vi "WeatherMapAPI_CurrentWeather-ParseResponseJSON.vi"(11 "API JSON Response":string) -> (3 "WeatherMap Current Weather Data":T1)   [LabVIEW 2021]
panel:
  out "Array":string[](array[string])
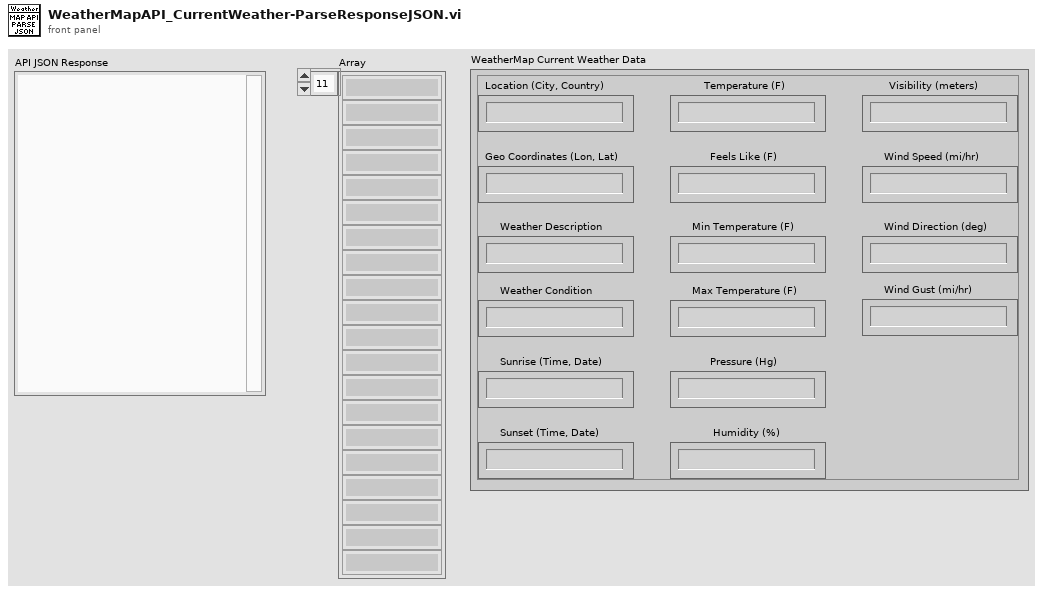
[diagram p1: front panel]
types:
  T1 = cluster{"Location (City, Country)":string, "Geo Coordinates (Lon, Lat)":string, "Weather Description ":string, "Weather Condition":string, "Temperature (F)":string, "Feels Like (F)":string, "Min Temperature (F)":string, "Max Temperature (F)":string, "Pressure (Hg) ":string, "Humidity (%)":string, "Visibility (meters)":string, "Wind Speed (mi/hr)":string, "Wind Direction (deg)":string, "Sunrise (Time, Date)":string, "Sunset (Time, Date)":string, "Wind Gust (mi/hr) ":string}
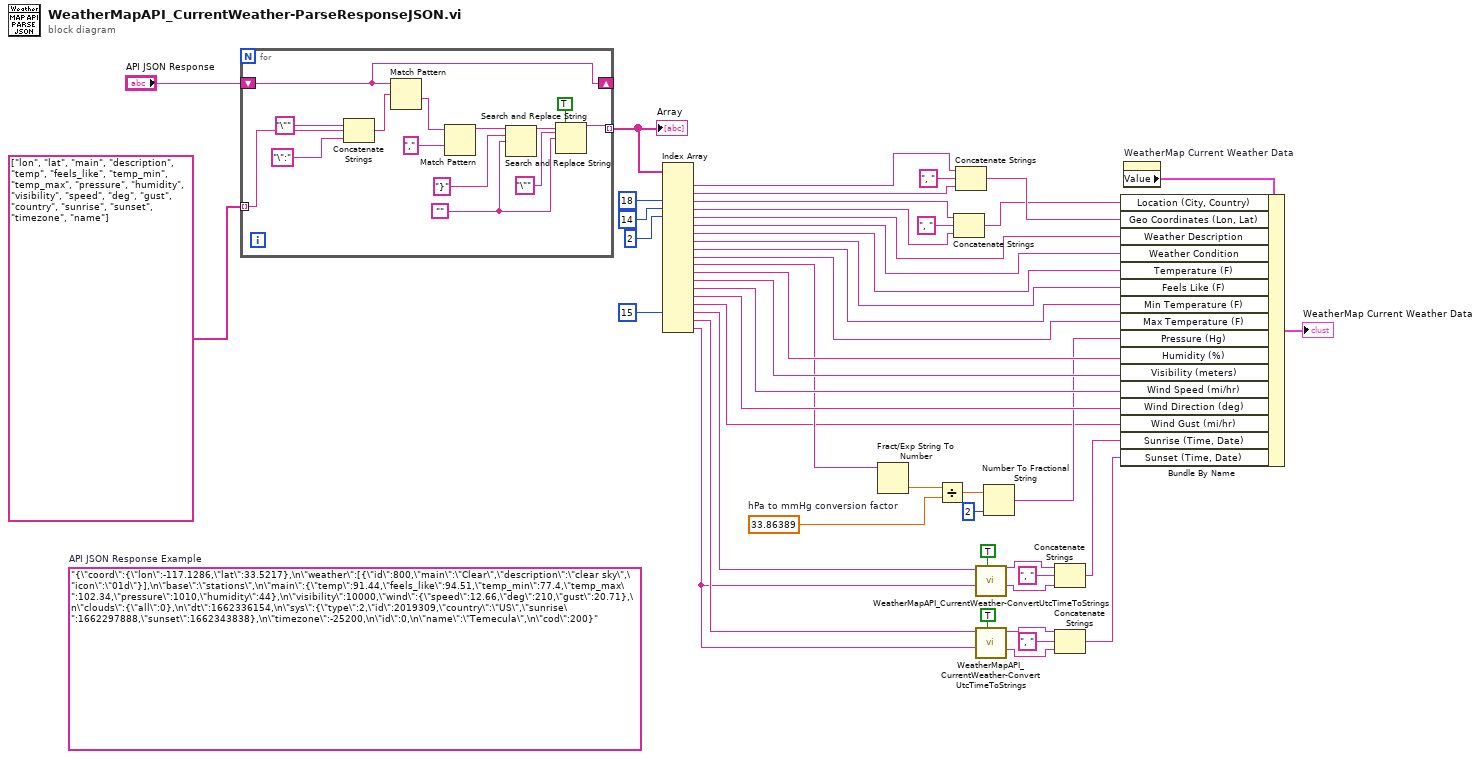
[diagram p0: block diagram]
diagram:
  w13 = 33.86389  # hPa to mmHg conversion factor
  (unwired) "{\"coord\":{\"lon\":-117.1286,\"lat\":33.5217},\n\"weather\":[{\"id\":800,\"main\":\"Clear\",\"description\":\"clear sky\",\"icon\":\"01d\"}],\n\"base\":\"stations\",\n\"main\":{\"temp\":91.44,\"feels_like\":94.51,\"temp_min\":77.4,\"temp_max\":102.34,\"pressure\":1010,\"humidity\":44},\n\"visibility\":10000,\"wind\":{\"speed\":12.66,\"deg\":210,\"gust\":20.71},\n\"clouds\":{\"all\":0},\n\"dt\":1662336154,\n\"sys\":{\"type\":2,\"id\":2019309,\"country\":\"US\",\"sunrise\":1662297888,\"sunset\":1662343838},\n\"timezone\":-25200,\n\"id\":0,\n\"name\":\"Temecula\",\n\"cod\":200}"  # API JSON Response Example
  n1 = for {
    shift-right: [w48] -> _
    shift-left: "API JSON Response" -> [w48]
    tunnel: string[] ["lon", "lat", "main", "description", "temp", "feels_like", "temp_min", "temp_max", "pressure", "humidity", "visibility", "speed", "deg", "gust", "country", "sunrise", "sunset", "timezone", "name"] -> [w58] mode=indexing
    tunnel: [w50] -> w45 mode=indexing
    w53 = ""
    n2 = Concatenate Strings("\"" ("regular expression"), w58, "\":" ("regular expression")) -> (w57:string)
    n3 = Match Pattern(string=w48, regular expression=w57) -> (after substring=w49:string)  [unwired: 1 in, 3 out]
    n4 = Match Pattern(string=w49, regular expression=",") -> (before substring=w55:string)  [unwired: 1 in, 3 out]
    n5 = Search and Replace String(input string=w55, search string="}", replace string=w53) -> (result string=w54:string)  [unwired: 5 in, 3 out]
    n6 = Search and Replace String(replace all?=TRUE ("replace all? (F)"), input string=w54, search string="\"", replace string=w53) -> (result string=w50:string)  [unwired: 4 in, 3 out]
  }
  "Array" <- w45
  n7 = Index Array(array=w45, index #3=18 ("index"), index #4=14 ("index"), index #5=2 ("index"), index #17=15 ("index")) -> (element #1=w43:string, element #2=w42:string, element #3=w37:string, element #4=w36:string, element #5=w31:string, element #6=w30:string, element #7=w29:string, element #8=w28:string, element #9=w27:string, element #10=w26:string, element #11=w8:string, element #12=w25:string, element #13=w24:string, element #14=w23:string, element #15=w22:string, element #16=w5:string, element #17=w3:string, element #18=w2:string, element #19=w1:string)  [unwired: 15 in]
  n8 = Fract/Exp String To Number(string=w8) -> (number=w9:dbl)  [unwired: 3 in, 1 out]
  n9 = Divide(x=w9, y=w13) -> (x/y=w12:dbl)
  n10 = Concatenate Strings(w37, ", " ("regular expression"), w36) -> (w35:string)
  n11 = Concatenate Strings(w43, ", " ("regular expression"), w42) -> (w39:string)
  n12 = call "WeatherMapAPI_CurrentWeather-ConvertUtcTimeToStrings.vi"("1Hr Adjust - Subtract"=TRUE, "Offset from UTC"=w1, "Sunrise/Sunset time, unix, UTC"=w3) -> ("Date"=w18:string, "Time"=w17:string)  [unwired: 7 in]
  n13 = call "WeatherMapAPI_CurrentWeather-ConvertUtcTimeToStrings.vi"("1Hr Adjust - Subtract"=TRUE, "Offset from UTC"=w1, "Sunrise/Sunset time, unix, UTC"=w2) -> ("Date"=w14:string, "Time"=w15:string)  [unwired: 7 in]
  n14 = Number To Fractional String(number=w12, precision (6)=i16 2) -> (F-format string=w10:string)  [unwired: 2 in]
  n15 = Concatenate Strings(w17, ", " ("regular expression"), w18) -> (w6:string)
  n16 = Concatenate Strings(w15, ", " ("regular expression"), w14) -> (w7:string)
  n17 = property on="WeatherMap Current Weather Data" class="Clust (strict)"() -> ("Value"=w40:T1)  [unwired: 2 in, 2 out]
  n18 = Bundle By Name(cluster=w40, "Location (City, Country)"=w35, "Geo Coordinates (Lon, Lat)"=w39, "Weather Description"=w31, "Weather Condition"=w30, "Temperature (F)"=w29, "Feels Like (F)"=w28, "Min Temperature (F)"=w27, "Max Temperature (F)"=w26, "Pressure (Hg)"=w10, "Humidity (%)"=w25, "Visibility (meters)"=w24, "Wind Speed (mi/hr)"=w23, "Wind Direction (deg)"=w22, "Wind Gust (mi/hr)"=w5, "Sunrise (Time, Date)"=w6, "Sunset (Time, Date)"=w7) -> (→"WeatherMap Current Weather Data":T1)
